vi "Update Table Display.vi"(10 "Auton Sequence":T1[](array[typedef]), 11 "MulticolumnListbox in":refnum<vi>) -> ()   [LabVIEW 2017]
uses:
  Typedef/Single Sequence.ctl
  Typedef/Sequence Command.ctl
  Typedef/Plate Arrangement.ctl
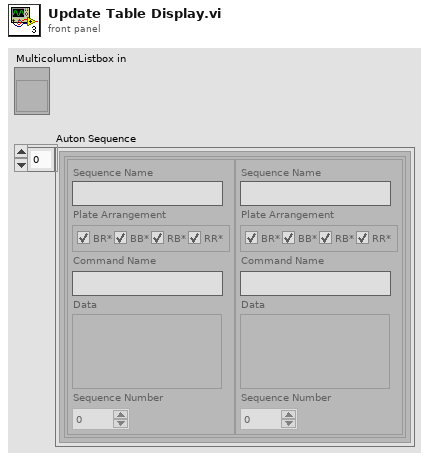
[diagram p1: front panel]
types:
  T1 = typedef "Single Sequence.ctl" = cluster{"Sequence Array":T2[]}
  T2 = typedef "Sequence Command.ctl" = cluster{"Sequence Name":string, "Plate Arrangement":T3, "Command Name":string, "Data":variant, "Sequence Number":u32}
  T3 = typedef "Plate Arrangement.ctl" = cluster{"BR*":bool, "BB*":bool, "RB*":bool, "RR*":bool}
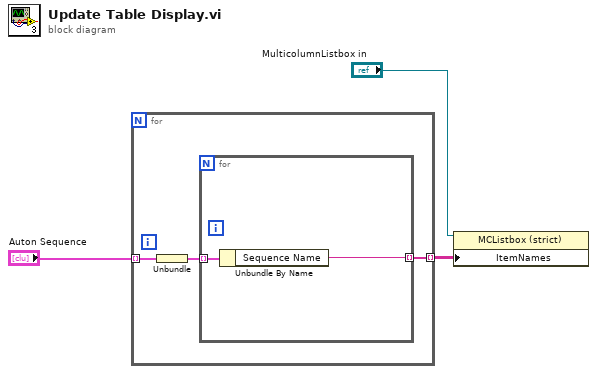
[diagram p0: block diagram]
diagram:
  n1 = for {
    tunnel: "Auton Sequence" -> [w6] mode=indexing
    tunnel: [w4] -> w2 mode=indexing
    n2 = Unbundle(w6) -> ("Sequence Array"=w5:T2[])
    n3 = for {
      tunnel: w5 -> [w8] mode=indexing
      tunnel: [w7] -> w4 mode=indexing
      n4 = Unbundle By Name(w8) -> ("Sequence Name"=w7:string)
    }
  }
  n5 = property class="MCListbox (strict)"(reference="MulticolumnListbox in", "ItemNames"=w2) -> ()  [unwired: 1 in, 2 out]
